vi "OpenMV_SelectROI.vi"(3 "image":picture) -> (0 "Rect":T1)   [LabVIEW 2017]
doc: "This VI pops up a window where the user can select a region of interest."
panel:
  in  "Pen":u32(colorbox)=16774656
  in  "ROI":T1
  out "Image":picture
  in  "OK":bool
  out "Display":picture caption="new picture"
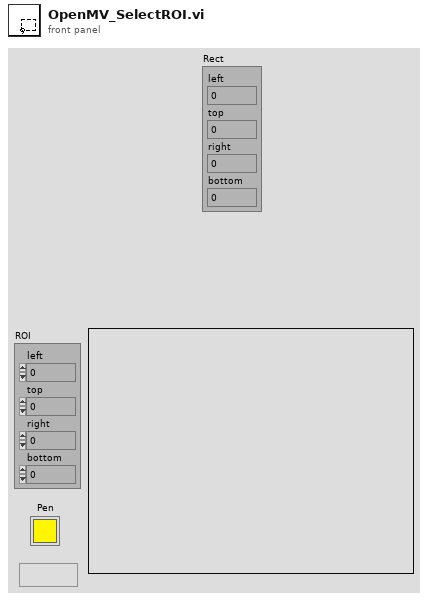
[diagram p1: front panel]
types:
  T1 = cluster{"left":i32, "top":i32, "right":i32, "bottom":i32}
  T2 = typedef "imagedata.ctl" = cluster{"image type":i32, "image depth":i32, "image":u8[], "mask":u8[], "colors":u32[], "Rectangle":cluster{"left":i16, "top":i16, "right":i16, "bottom":i16}}
  T3 = typedef "LVRectTypeDef.ctl" = cluster{"Left":i16, "Top":i16, "Right":i16, "Bottom":i16}
  T4 = cluster{"left":i16, "top":i16, "right":i16, "bottom":i16}
  T5 = typedef "LVMouseTypeDef.ctl" = cluster{"Mouse Position":cluster{"X":i32, "Y":i32}, "Mouse Modifiers":cluster{"Button Down":bool, "Shift Mod":bool, "Menu Mod":bool, "Option Mod":bool}}
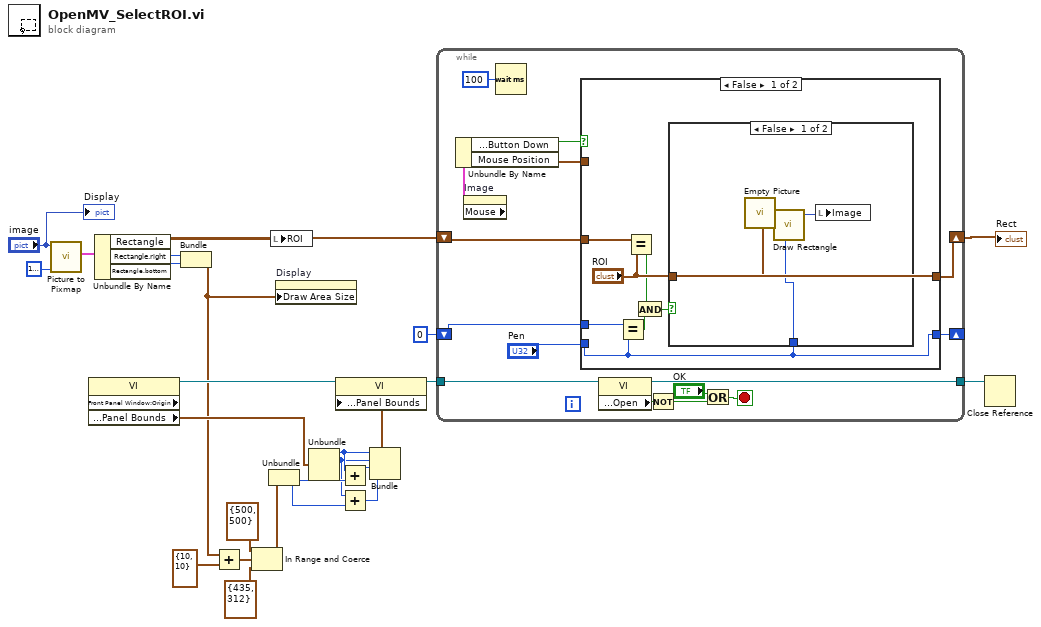
[diagram p0: block diagram]
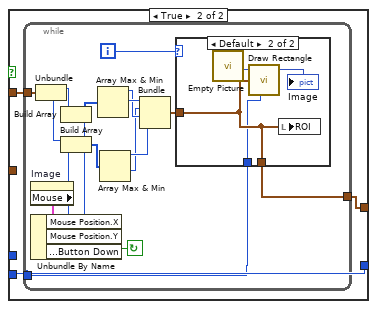
[diagram p3: hidden frame]
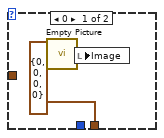
[diagram p4: hidden frame]
diagram:
  n1 = call <vilib>:"Picture to Pixmap.vi"("Background Color"=u32 16777216, "picture"="image") -> ("image data"=w8:T2)  [unwired: 8 in, 1 out]
  n2 = property class="VI" props=["Front Panel Window:Origin", "Front Panel Window:Panel Bounds"]() -> (reference out=w23:refnum<vi>, "Front Panel Window:Panel Bounds"=w20:T3)  [unwired: 2 in, 2 out]
  n3 = Unbundle By Name(w8) -> ("Rectangle"=w3:T4, "Rectangle.right"=w7:i16, "Rectangle.bottom"=w6:i16)
  n4 = Bundle("right"=w7, "bottom"=w6) -> (w5:cluster{"right":i16, "bottom":i16})  [unwired: 1 in]
  n5 = Add(x=w5, y=cluster{i32, i32} {10, 10} ("x+y")) -> (x+y=w11:cluster{i32, i32})
  n6 = In Range and Coerce(upper limit=cluster{i32, i32} {500, 500}, x=w11, lower limit=cluster{i32, i32} {435, 312} ("x+y")) -> (coerced(x)=w10:cluster{i32, i32})  [unwired: 1 out]
  n7 = Unbundle(w10) -> (w17:i32, w16:i32)
  n8 = local write "ROI"(w3) -> ()
  n9 = property on="Display" class="Pict"("Draw Area Size"=w5) -> ()  [unwired: 2 in, 2 out]
  n10 = Unbundle(w20) -> ("Left"=w15:i16, "Top"=w14:i16)  [unwired: 2 out]
  n11 = Add(x=w15, y=w17) -> (x+y=w19:i32)
  n12 = Add(x=w14, y=w16) -> (x+y=w18:i32)
  n13 = Bundle("Left"=w15, "Top"=w14, w19, w18) -> (w21:cluster{"Left":i16, "Top":i16, i32, i32})  [unwired: 1 out]
  n14 = property class="VI"(reference=w23, "Front Panel Window:Panel Bounds"=w21) -> (reference out=w1:refnum<vi>)  [unwired: 1 in, 1 out]
  n15 = while {
    shift-left: u32 0 ("Pen") -> [w26]
    shift-right: [w28] -> _
    shift-left: w3 -> [w30]
    shift-right: [w31] -> w24
    tunnel: [w27] -> w25
    tunnel: w1 -> [w37]
    stop <- w33 stop-if-true
    n16 = property on="Image" class="Pict"() -> ("Mouse"=w40:T5)  [unwired: 2 in, 2 out]
    n17 = Unbundle By Name(w40) -> ("Mouse Modifiers.Button Down"=w32:bool, "Mouse Position"=w39:cluster{"X":i32, "Y":i32})
    n18 = Wait (ms)(milliseconds to wait=u32 100) -> ()  [unwired: 1 out]
    n19 = case shown="False" w32 {
      tunnel: w39 -> [_ w54]
      tunnel: ["ROI" w53] -> w31
      tunnel: w30 -> [w47 _]
      tunnel: "Pen" -> [w44 w52]
      tunnel: [w44 w52] -> w28
      tunnel: w26 -> [w45 _]
      frame False {
        n20 = Equal?(x=w45, y=w44) -> (x = y?=w43:bool)
        n21 = Equal?(x=w47, y="ROI") -> (x = y?=w42:bool)
        n22 = And(x=w42, y=w43) -> (x .and. y?=w41:bool)
        n23 = case shown="False" w41 {
          tunnel: "ROI" -> [w49 _]
          tunnel: w44 -> [w50 _]
          frame False {
            n24 = call "Empty Picture"() -> ("empty picture"=w51:picture)
            n25 = call <vilib>:"Draw Rectangle.vi"("picture"=w51, "rect"=w49, "color(black)"=w50) -> ("new picture"=w48:picture)  [unwired: 6 in]
            n26 = local write "Image"(w48) -> ()
          }
          frame True {
          }
        }
      }
      frame True {
        n27 = while {
          tunnel: w52 -> [w55]
          tunnel: [w56] -> w53
          tunnel: w54 -> [w68]
          i -> [w71]
          stop <- w69 continue-if-true
          n28 = property on="Image" class="Pict"() -> ("Mouse"=w70:T5)  [unwired: 2 in, 2 out]
          n29 = Unbundle By Name(w70) -> ("Mouse Position.X"=w66:i32, "Mouse Position.Y"=w64:i32, "Mouse Modifiers.Button Down"=w69:bool)
          n30 = Unbundle(w68) -> ("X"=w67:i32, "Y"=w65:i32)
          n31 = Build Array(w67, w66) -> (w63:i32[])
          n32 = Build Array(w65, w64) -> (w60:i32[])
          n33 = Array Max & Min(array=w63) -> (max value=w61:i32, min value=w62:i32)  [unwired: 2 out]
          n34 = Array Max & Min(array=w60) -> (max value=w59:i32, min value=w58:i32)  [unwired: 2 out]
          n35 = Bundle(w62, w58, w61, w59) -> (w57:cluster{i32, i32, i32, i32})  [unwired: 1 out]
          n36 = case shown="Default" w71 {
            tunnel: w57 -> [_ w77]
            tunnel: [cluster{i32, i32, i32, i32} {0, 0, 0, 0} w77] -> w56
            tunnel: w55 -> [_ w74]
            frame 0 {
              n37 = call "Empty Picture"() -> ("empty picture"=w73:picture)
              n38 = local write "Image"(w73) -> ()
            }
            frame Default {
              n39 = call "Empty Picture"() -> ("empty picture"=w76:picture)
              n40 = call <vilib>:"Draw Rectangle.vi"("picture"=w76, "rect"=w77, "color(black)"=w74) -> ("new picture"=→"Image":picture)  [unwired: 6 in]
              n41 = local write "ROI"(w77) -> ()
            }
          }
        }
      }
    }
    n42 = property class="VI"(reference=w37) -> (reference out=w27:refnum<vi>, "Front Panel Window:Open"=w36:bool)  [unwired: 1 in, 1 out]
    n43 = Not(x=w36) -> (.not. x?=w34:bool)
    n44 = Or(x="OK", y=w34) -> (x .or. y?=w33:bool)
  }
  "Rect" <- w24
  n45 = Close Reference(reference=w25) -> ()  [unwired: 1 in, 1 out]
  "Display" <- "image"
